vi "V to moisture converter.vi"(1 "Waveform":dbl) -> (0 "Numeric":dbl)   [LabVIEW 2022 SP3]
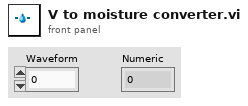
[diagram p1: front panel]
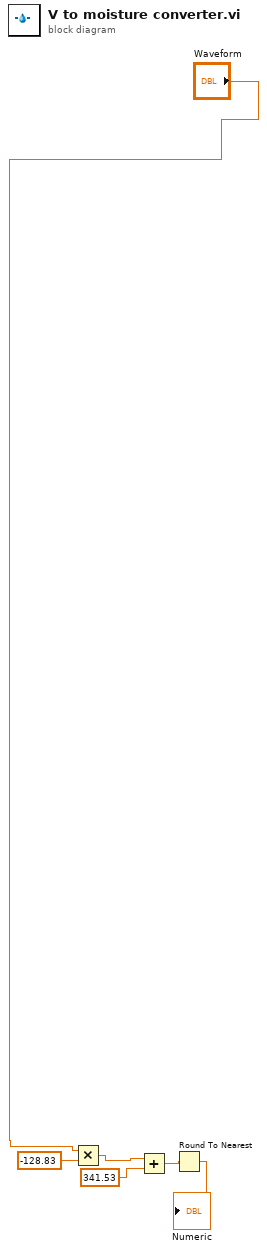
[diagram p0: block diagram]
diagram:
  n1 = Multiply(x="Waveform", y=-128.83) -> (x*y=w4:dbl)
  n2 = Add(x=w4, y=341.53) -> (x+y=w5:dbl)
  n3 = Round To Nearest(number=w5) -> (nearest integer value=→"Numeric":dbl)
